vi "Message type.vi"(11 "IWampMessage in":refnum<class "IWampMessage.lvclass">) -> (2 "Message Codes":T1, 3 "IWampMessage out":refnum<class "IWampMessage.lvclass">)   [LabVIEW 2020, in "wamplv.lvlib" / "IWampMessage.lvclass"]
uses:
  IWampMessage.lvclass
  TypeDefs/WAMP Message Codes.ctl
  wamplv.lvlib
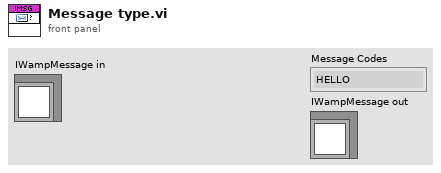
[diagram p1: front panel]
types:
  T1 = typedef "wamplv.lvlib/WAMP Message Codes.ctl" = enum8{"HELLO", "WELCOME", "ABORT", "GOODBYE", "ERROR", "PUBLISH", "PUBLISHED", "SUBSCRIBE", "SUBSCRIBED", "UNSUBSCRIBE", "UNSUBSCRIBED", "EVENT", "CALL", "RESULT", "REGISTER", "REGISTERED", "UNREGISTER", "UNREGISTERED", "INVOCATION", "YIELD"}
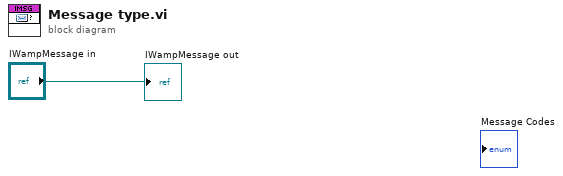
[diagram p0: block diagram]
diagram:
  "IWampMessage out" <- "IWampMessage in"
